vi "Daten speichern auf PC Dateien.vi"(7 "IP Adresse":string, 8 "error in":errorcluster, 10 "Dateinamen":string[](array[string]), 11 "Pfad PC":path caption="Lokaler Pfad") -> (0 "error out":errorcluster, 2 "ohne Fehler":bool)   [LabVIEW 2020, in "FTP WebDAV.lvlib"]
uses:
  FTP WebDAV.lvlib
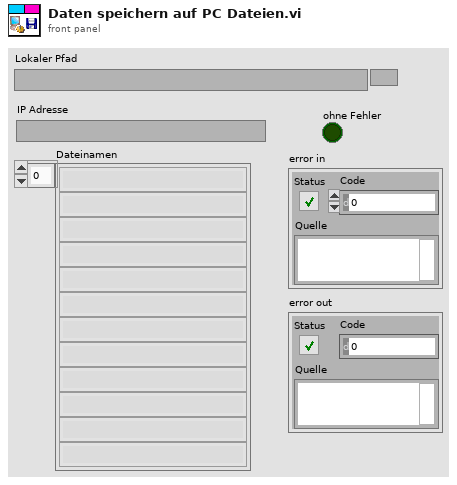
[diagram p1: front panel]
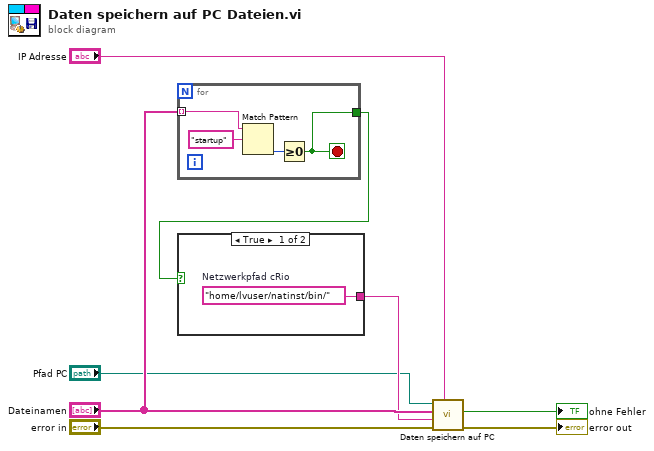
[diagram p0: block diagram]
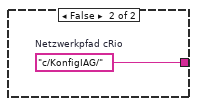
[diagram p2: hidden frame]
diagram:
  n1 = for {
    tunnel: "Dateinamen" -> [w10] mode=indexing
    tunnel: [w9] -> w8
    stop <- w9 stop-if-true
    n2 = Match Pattern(string=w10, regular expression="startup" ("Regulärer Ausdruck")) -> (offset past match=w12:i32)  [unwired: 1 in, 3 out]
    n3 = Greater Or Equal To 0?(x=w12) -> (x >= 0?=w9:bool)
  }
  n4 = case shown="True" w8 {
    tunnel: [w13 w14] -> w5
    frame True {
      w13 = "home/lvuser/natinst/bin/"  # Netzwerkpfad cRio
    }
    frame False {
      w14 = "c/KonfigIAG/"  # Netzwerkpfad cRio
    }
  }
  n5 = call "Daten speichern auf PC.vi"("IP Adresse"="IP Adresse", "error in"="error in", "Pfad PLC"=w5, "Dateinamen"="Dateinamen", "Pfad PC"="Pfad PC") -> ("error out"=→"error out":errorcluster, "ohne Fehler"=→"ohne Fehler":bool)  [unwired: 4 in, 1 out]
